vi "RoomsFGVLocalErrorH.vi"(8 "error in (no error)":errorcluster, 11 "String in":string) -> (0 "error out":errorcluster, 3 "String out":string)   [LabVIEW 2015]
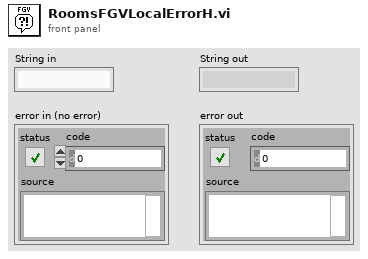
[diagram p1: front panel]
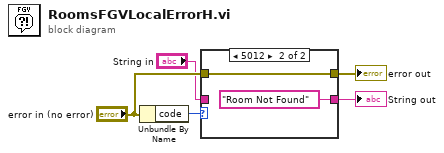
[diagram p0: block diagram]
diagram:
  n1 = Unbundle By Name("error in (no error)") -> ("code"=w1:i32)
  n2 = case shown="5012" w1 {
    tunnel: [w7 "Room Not Found" ("String")] -> w5
    tunnel: [w6 w8] -> w3
    tunnel: "error in (no error)" -> [w6 w8]
    tunnel: "String in" -> [w7 _]
    frame 0, Default {
    }
    frame 5012 {
    }
  }
  "error out" <- w3
  "String out" <- w5
